vi "CONST AI RawDataQ KeyName.vi"(4 "Select":T1, 6 "AI TaskName":string) -> (7 "AI RawDataQ (KeyName)":string)   [LabVIEW 2017, in "DAQ.lvclass"]
doc: "Developed by Kevin Thompson\nkevin@thompsonengineering.net\n\nCopyright 2018-2020\nThompson Engineering, LLC"
uses:
  DAQ.lvclass
  DataTypes/TD AI RawDataQ SelectType--enum.ctl
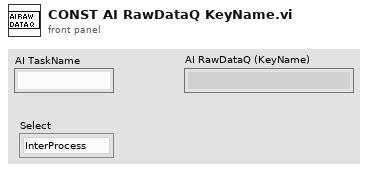
[diagram p1: front panel]
types:
  T1 = typedef "DAQ.lvclass/TD AI RawDataQ SelectType--enum.ctl" = enum16{"InterProcess", "LocalDAQThread"}
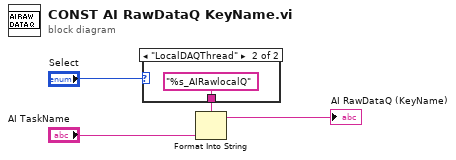
[diagram p0: block diagram]
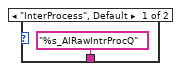
[diagram p2: hidden frame]
diagram:
  n1 = case shown="\"LocalDAQThread\"" "Select" {
    tunnel: ["%s_AIRawIntrProcQ" ("format string") "%s_AIRawlocalQ" ("format string")] -> w1
    frame "InterProcess", Default {
    }
    frame "LocalDAQThread" {
    }
  }
  n2 = Format Into String(format string=w1, "AI TaskName") -> (resulting string=→"AI RawDataQ (KeyName)":string)  [unwired: 2 in, 1 out]
